vi "Provera mase (SubVI).vi"(2 "Waveform":dbl, 3 "Opis predmeta":T1) -> (0 "masa":dbl, 1 "Boolean":bool)   [LabVIEW 2017]
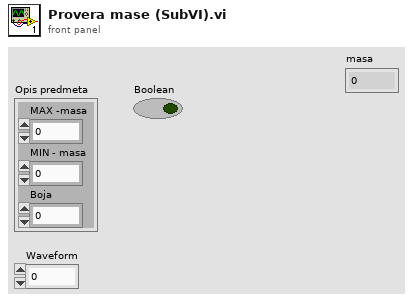
[diagram p1: front panel]
types:
  T1 = cluster{"MAX -masa":dbl, "MIN - masa":dbl, "Boja":u32}
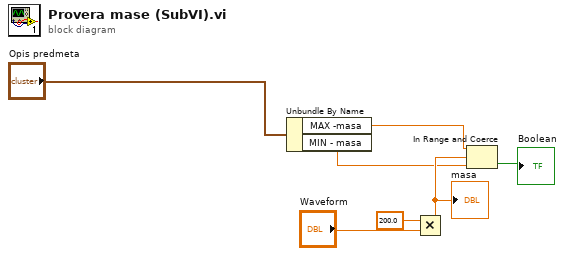
[diagram p0: block diagram]
diagram:
  n1 = Unbundle By Name("Opis predmeta") -> ("MAX -masa"=w3:dbl, "MIN - masa"=w4:dbl)
  n2 = Multiply(x=200.0, y="Waveform") -> (x*y=w7:dbl)
  "masa" <- w7
  n3 = In Range and Coerce(upper limit=w3, x=w7, lower limit=w4) -> (In Range?=→"Boolean":bool)  [unwired: 1 out]
